vi "H5Pget_chunk.vi"(6 "error in (no error)":errorcluster, 9 "HDF5 Property Ref":T1) -> (0 "error out":errorcluster, 2 "Dimensions":u64[](array[numeric]), 3 "HDF5 Ref out":T1)   [LabVIEW 2017]
doc: "Retrieves the size of chunks for the raw data of a chunked layout dataset."
uses:
  <vilib>/UPVI/lvhdf5/library.llb/HDF5 Ref.ctl
  <vilib>/UPVI/lvhdf5/hdf5.dll
panel:
  # "LVHDF5 Toolkit\nCopyright (c) 2005-2013 by Jason D. Sommerville\nCopyright (c) 2014 by UPVI, LLC.\n\nThis use and distribution of this file is governed by the terms found in \nLICENSE.txt distributed with this toolkit and installed at\n <user.lib>\\_lvhdf5\\LICENSE.txt"
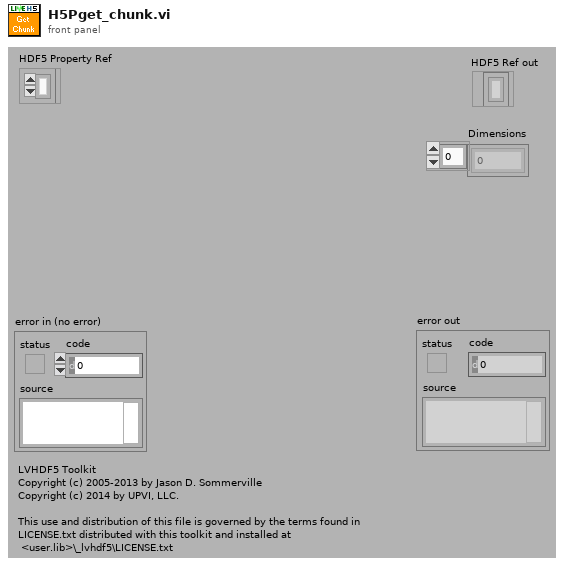
[diagram p1: front panel]
types:
  T1 = typedef "HDF5 Ref.ctl" = refnum<k1>
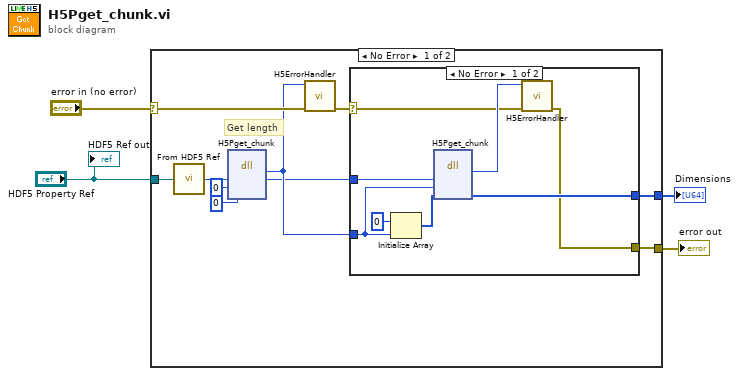
[diagram p0: block diagram]
diagram:
  n1 = case shown="No Error" "error in (no error)" {
    selector: "error in (no error)" -> [w9 w24]
    tunnel: [w14 w24] -> w3
    tunnel: "HDF5 Property Ref" -> [w13 _]
    tunnel: [w5 _] -> w1
    frame No Error {
      # "Get length"
      n2 = call <vilib>:"From HDF5 Ref.vi"("HDF5 Ref"=w13) -> ("I32"=w12:i32)
      n3 = dll-call lib="C:/Program Files/National Instruments/LabVIEW 2017/vi.lib/UPVI/lvhdf5/hdf5.dll" fn="H5Pget_chunk"("plist_id"=w12, "ndims"=0, "dim"=u32 0) -> (w8:i32, "plist_id"=w6:i32)  [unwired: 5 in, 2 out]
      n4 = call <vilib>:"H5ErrorHandler.vi"("error in (no error)"=w9, "herr_t"=w8) -> ("error out"=w7:errorcluster)  [unwired: 3 in, 4 out]
      n5 = case shown="No Error" w7 {
        selector: w7 -> [w21 w23]
        tunnel: [w15 w23] -> w14
        tunnel: w8 -> [w18 _]
        tunnel: w6 -> [w17 _]
        tunnel: [w16 _] -> w5
        frame No Error {
          n6 = Initialize Array(u64 0, w18) -> (w19:u64[])
          n7 = dll-call lib="C:/Program Files/National Instruments/LabVIEW 2017/vi.lib/UPVI/lvhdf5/hdf5.dll" fn="H5Pget_chunk"("plist_id"=w17, "ndims"=w18, "dim"=w19) -> ("return type"=w22:i32, "dim"=w16:u64[])  [unwired: 5 in, 2 out]
          n8 = call <vilib>:"H5ErrorHandler.vi"("error in (no error)"=w21, "herr_t"=w22) -> ("error out"=w15:errorcluster)  [unwired: 3 in, 4 out]
        }
        frame Error {
        }
      }
    }
    frame Error {
    }
  }
  "error out" <- w3
  "Dimensions" <- w1
  "HDF5 Ref out" <- "HDF5 Property Ref"
